vi "SaveMSR_SRSI.vi"(8 "error in (no error)":errorcluster, 9 "SRSI Parameters":T1={"sensitivity"=0.11032028469750889, "Filter"={"Tau (fs)"=9.75e-13, "fwhm (fs)"=3.2551150895140684e-13, "filter gaussian power"=30}, "Poly Fit Order"=4, "N XPW Loop"=3, "Scales Unit"=enum."nm", "Results average"=0, "Spectral filter"={"min"=0.0, "max"=0.0, "Level"=0.0}, "Apodization"={"Auto"=TRUE, "WL min"=6.000000000000001e-07, "WL max"=1.0000000000000002e-06}, "Warning levels"={"Min level"=5000.0, "Max level"=62000.0, "Min contrast"=0.1}, "NormXPW"=FALSE, "DisableChecks"=FALSE, "External\nFund. Spectrum"=FALSE, "XPW factors"={"Optimize"=enum."Never", "Blue Shift Correction"=0.0, "Parasite Amp"=0.0}}, 10 "RAW SRSI Spectrum":T2, 11 "MSR path":path caption="selected path") -> (0 "error out":errorcluster, 3 "dup. MSR path":path)   [LabVIEW 2020]
uses:
  SRSI_Parameters.ctl
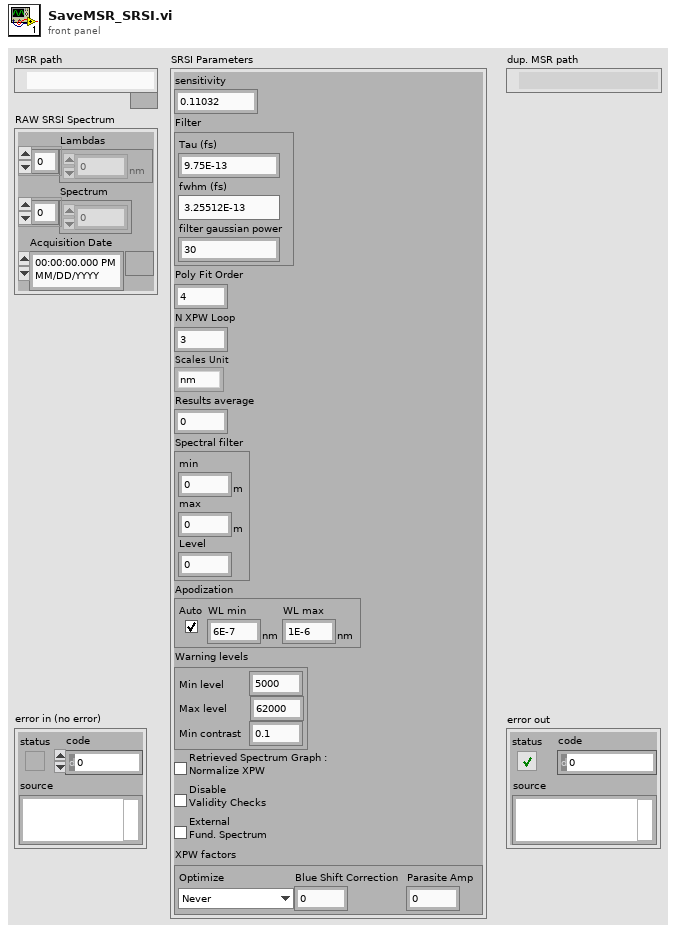
[diagram p1: front panel]
types:
  T1 = typedef "SRSI_Parameters.ctl" = cluster{"sensitivity":dbl, "Filter":cluster{"Tau (fs)":dbl[unit], "fwhm (fs)":dbl[unit], "filter gaussian power":i32}, "Poly Fit Order":i32, "N XPW Loop":u16, "Scales Unit":enum16{"nm", "THz", "cm^-1"}, "Results average":i32, "Spectral filter":cluster{"min":dbl[unit], "max":dbl[unit], "Level":dbl}, "Apodization":cluster{"Auto":bool, "WL min":dbl[unit], "WL max":dbl[unit]}, "Warning levels":cluster{"Min level":dbl, "Max level":dbl, "Min contrast":dbl}, "NormXPW":bool, "DisableChecks":bool, "External\nFund. Spectrum":bool, "XPW factors":cluster{"Optimize":enum16{"Never", "Once", "Ever"}, "Blue Shift Correction":dbl, "Parasite Amp":dbl}}
  T2 = cluster{"Lambdas":sgl[unit][], "Spectrum":sgl[], "Acquisition Date":timestamp}
  T3 = enum16{"Get Variant Array From Measure", "Set Measure From Variant Array"}
  T4 = cluster{"Measure Type":string, "Date":string, "Time":string, "Parameters (Variant)":variant[], "Lambdas":sgl[unit][], "Raw spectra":sgl[][]}
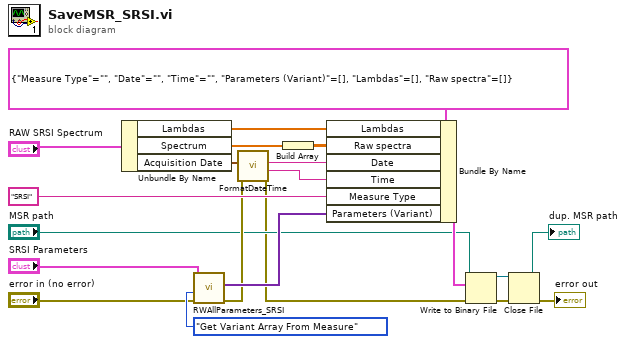
[diagram p0: block diagram]
diagram:
  n1 = Unbundle By Name("RAW SRSI Spectrum") -> ("Lambdas"=w18:sgl[unit][], "Spectrum"=w17:sgl[], "Acquisition Date"=w15:timestamp)
  n2 = call "RWAllParameters_SRSI.vi"("error in (no error)"="error in (no error)", "Read/Write"=T3."Get Variant Array From Measure", "Parameters In"="SRSI Parameters") -> ("error out"=w11:errorcluster, "Parameters Out"=w12:variant[])  [unwired: 6 in, 1 out]
  n3 = call "FormatDateTime.vi"("error in"=w11, "Unformatted  Date"=w15) -> ("error out"=w2:errorcluster, "Time"=w13:string, "Date"=w14:string)  [unwired: 7 in]
  n4 = Build Array(w17) -> (w6:sgl[][])
  n5 = Bundle By Name(cluster=T4 {"Measure Type"="", "Date"="", "Time"="", "Parameters (Variant)"=[], "Lambdas"=[], "Raw spectra"=[]}, "Lambdas"=w18, "Raw spectra"=w6, "Date"=w14, "Time"=w13, "Measure Type"="SRSI", "Parameters (Variant)"=w12) -> (w19:T4)
  n6 = Write to Binary File(file (use dialog)="MSR path", data=w19, error in=w2) -> (refnum out=w3:refnum<file>, error out=w4:errorcluster)  [unwired: 3 in, 1 out]
  n7 = Close File(refnum=w3, error in=w4) -> (path=→"dup. MSR path":path, error out=→"error out":errorcluster)
